vi "getHWConfig.vi"(8 "error in (no error)":errorcluster, 11 "HWConfiguration in":refnum<class "HWConfiguration.lvclass">) -> (0 "error out":errorcluster, 3 "HWConfiguration out":refnum<class "HWConfiguration.lvclass">)   [LabVIEW 2009, in "Hardware.lvlib" / "HWControllers.lvlib" / "HWConfiguration.lvclass"]
uses:
  HWConfiguration.lvclass
  HWConfiguration.lvclass/HWConfiguration.ctl
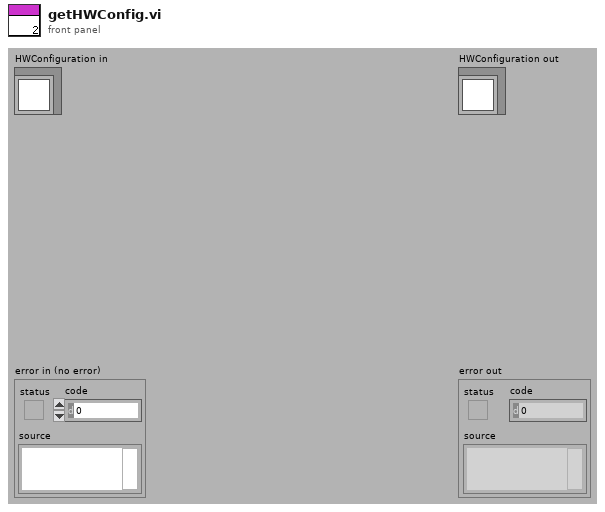
[diagram p1: front panel]
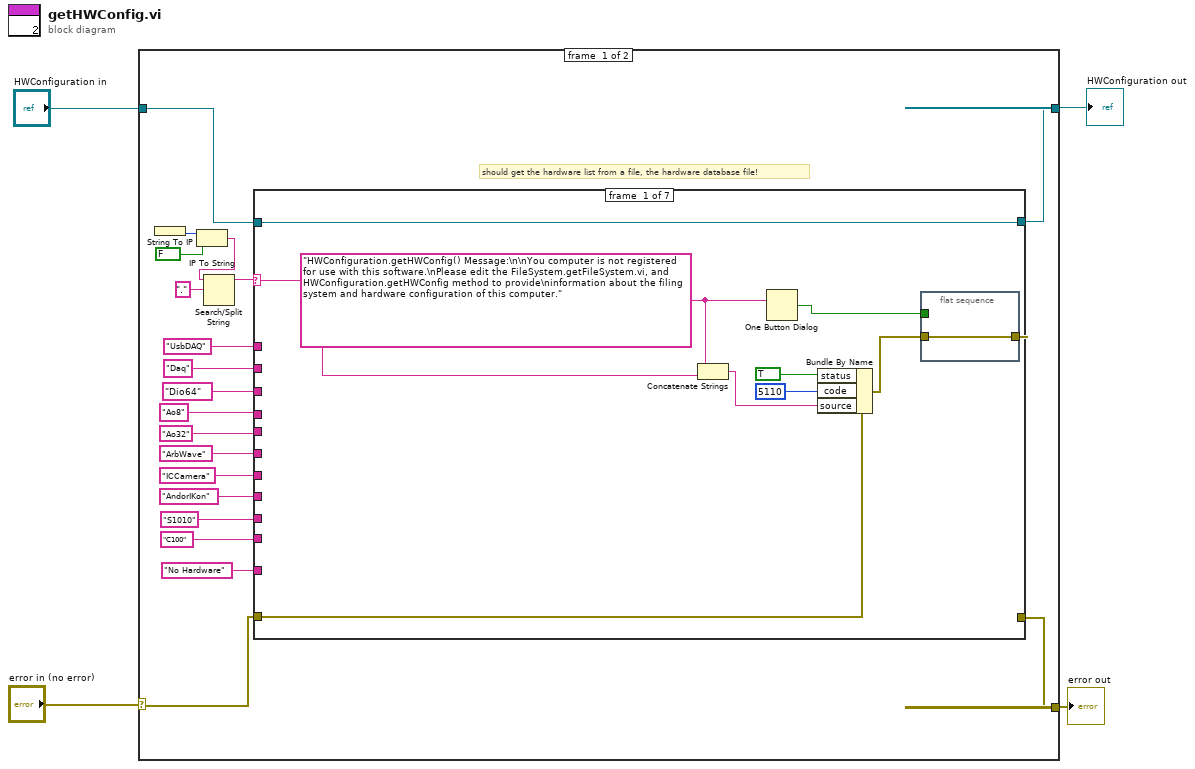
[diagram p0: block diagram]
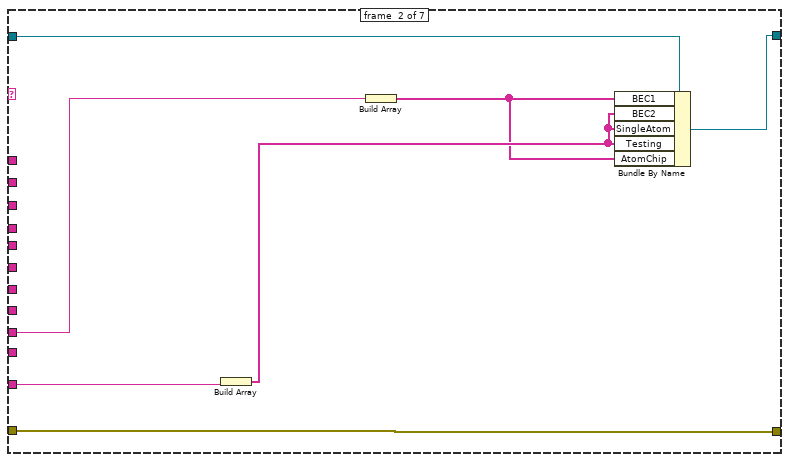
[diagram p2: hidden frame]
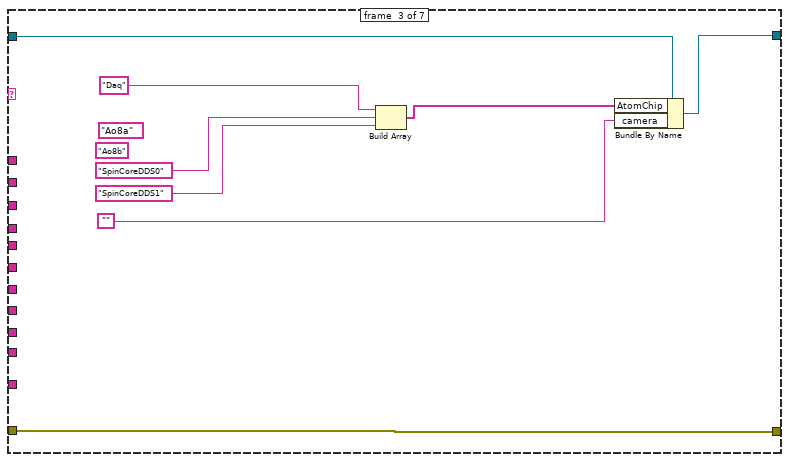
[diagram p3: hidden frame]
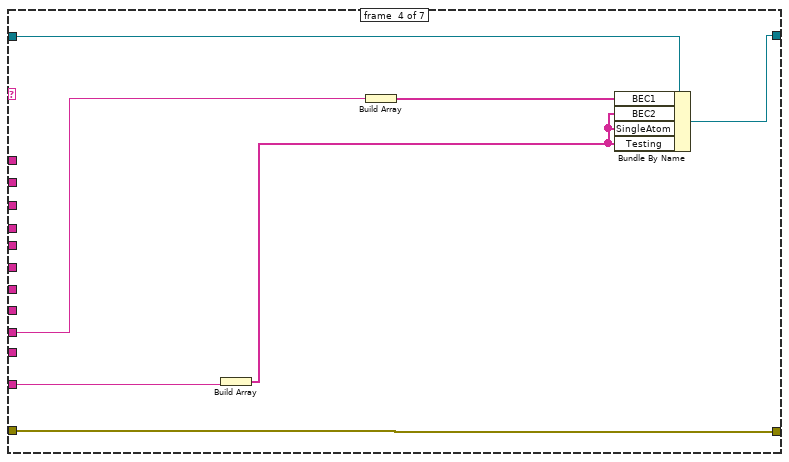
[diagram p4: hidden frame]
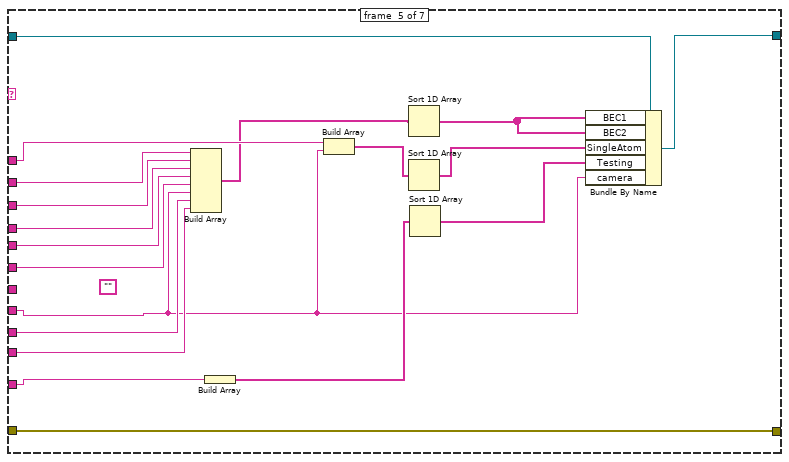
[diagram p5: hidden frame]
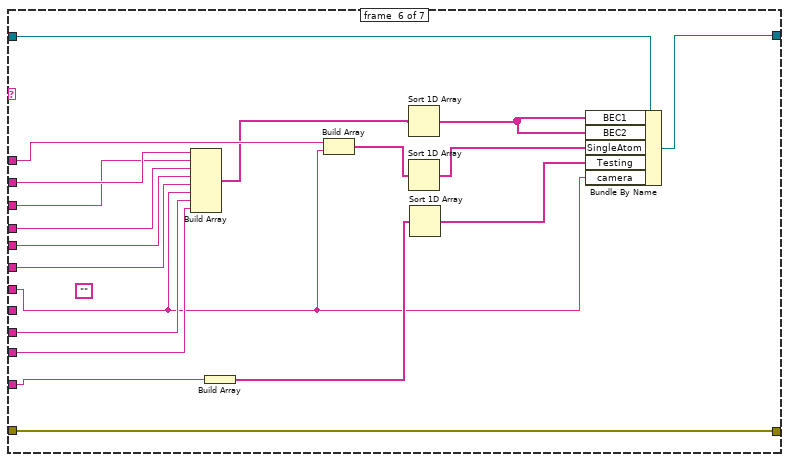
[diagram p6: hidden frame]
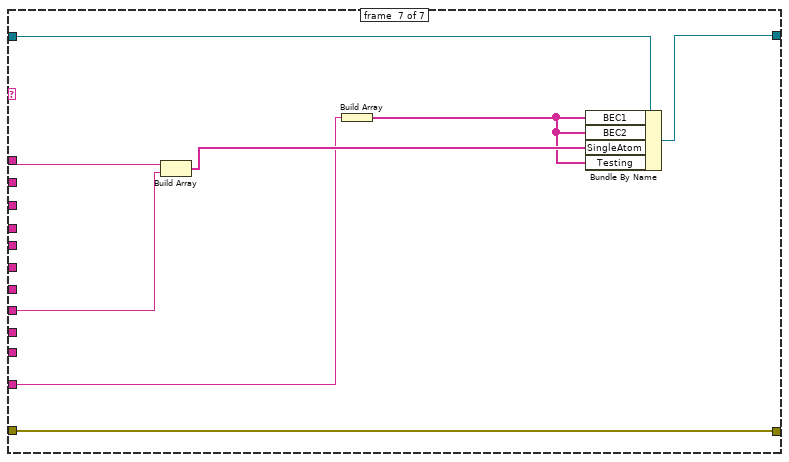
[diagram p7: hidden frame]
diagram:
  n1 = case shown="No Error" "error in (no error)" {
    selector: "error in (no error)" -> [w19 w105]
    tunnel: [w16 w105] -> w3
    tunnel: [w17 w104] -> w1
    tunnel: "HWConfiguration in" -> [w18 w104]
    frame #0 {
      # "should get the hardware list from a file, the hardware database file!"
      n2 = String To IP() -> (0:w23:u32)  [unwired: 1 in]
      n3 = IP To String(1:FALSE, 2:w23) -> (0:w21:string)
      n4 = Search/Split String(string=w21, search string/char (-)=".") -> (substring before match=w20:string)  [unwired: 1 in, 2 out]
      n5 = case shown="\"FCTX52S\"" w20 {
        selector: w20 -> [w28 _ _ _ _ _ _]
        tunnel: w18 -> [w25 w41 w49 w56 w75 w94 w102]
        tunnel: [w25 w40 w48 w55 w74 w93 w101] -> w17
        tunnel: w19 -> [w26 w42 w50 w57 w76 w95 w103]
        tunnel: [w31 w42 w50 w57 w76 w95 w103] -> w16
        tunnel: "UsbDAQ" -> [_ _ _ _ w66 w85 w100]
        tunnel: "Daq" -> [_ _ _ _ w73 w92 _]
        tunnel: "Dio64" -> [_ _ _ _ w59 w77 _]
        tunnel: "Ao8" -> [_ _ _ _ w72 w91 _]
        tunnel: "Ao32" -> [_ _ _ _ w71 w90 _]
        tunnel: "ArbWave" -> [_ _ _ _ w70 w89 _]
        tunnel: "ICCamera" -> [_ _ _ _ _ w78 _]
        tunnel: "AndorIKon" -> [_ _ _ _ w58 _ w99]
        tunnel: "S1010" -> [_ w37 _ w52 w69 w88 _]
        tunnel: "C100" -> [_ _ _ _ w68 w87 _]
        tunnel: "No Hardware" -> [_ w39 _ w54 w67 w86 w96]
        frame #0 {
          w29 = "HWConfiguration.getHWConfig() Message:\n\nYou computer is not registered for use with this software.\nPlease edit the FileSystem.getFileSystem.vi, and HWConfiguration.getHWConfig method to provide\ninformation about the filing system and hardware configuration of this computer."
          n6 = Concatenate Strings(w29, w28) -> (w27:string)
          n7 = One Button Dialog(message=w29) -> (true=w30:bool)  [unwired: 1 in]
          n8 = Bundle By Name(cluster=w26, "status"=TRUE, "code"=5110, "source"=w27) -> (w32:errorcluster)
          n9 = flat-sequence {
            tunnel: w32 -> [w35]
            tunnel: [w35] -> w31
            tunnel: w30 -> [_]
            frame #0 {
            }
          }
        }
        frame #1 {
          n10 = Build Array(w39) -> (w38:string[])
          n11 = Build Array(w37) -> (w36:string[])
          n12 = Bundle By Name(cluster=w41, "BEC1"=w36, "BEC2"=w38, "SingleAtom"=w38, "Testing"=w38, "AtomChip"=w36) -> (w40:refnum<class "HWConfiguration.lvclass">)
        }
        frame #2 {
          (unwired) "Ao8b"
          (unwired) "Ao8a"
          n13 = Build Array("Daq", "SpinCoreDDS0", "SpinCoreDDS1") -> (w45:string[])
          n14 = Bundle By Name(cluster=w49, "AtomChip"=w45, "camera"="") -> (w48:refnum<class "HWConfiguration.lvclass">)
        }
        frame #3 {
          n15 = Build Array(w54) -> (w53:string[])
          n16 = Build Array(w52) -> (w51:string[])
          n17 = Bundle By Name(cluster=w56, "BEC1"=w51, "BEC2"=w53, "SingleAtom"=w53, "Testing"=w53) -> (w55:refnum<class "HWConfiguration.lvclass">)
        }
        frame #4 {
          (unwired) ""
          n18 = Build Array(w73, w59, w72, w71, w70, w58, w69, w68) -> (w65:string[])
          n19 = Build Array(w67) -> (w61:string[])
          n20 = Build Array(w66, w58) -> (w63:string[])
          n21 = Sort 1D Array(array=w65) -> (sorted array=w64:string[])
          n22 = Sort 1D Array(array=w63) -> (sorted array=w62:string[])
          n23 = Sort 1D Array(array=w61) -> (sorted array=w60:string[])
          n24 = Bundle By Name(cluster=w75, "BEC1"=w64, "BEC2"=w64, "SingleAtom"=w62, "Testing"=w60, "camera"=w58) -> (w74:refnum<class "HWConfiguration.lvclass">)
        }
        frame #5 {
          (unwired) ""
          n25 = Build Array(w92, w77, w91, w90, w89, w78, w88, w87) -> (w84:string[])
          n26 = Build Array(w86) -> (w80:string[])
          n27 = Build Array(w85, w78) -> (w82:string[])
          n28 = Sort 1D Array(array=w84) -> (sorted array=w83:string[])
          n29 = Sort 1D Array(array=w82) -> (sorted array=w81:string[])
          n30 = Sort 1D Array(array=w80) -> (sorted array=w79:string[])
          n31 = Bundle By Name(cluster=w94, "BEC1"=w83, "BEC2"=w83, "SingleAtom"=w81, "Testing"=w79, "camera"=w78) -> (w93:refnum<class "HWConfiguration.lvclass">)
        }
        frame #6 {
          n32 = Build Array(w100, w99) -> (w98:string[])
          n33 = Build Array(w96) -> (w97:string[])
          n34 = Bundle By Name(cluster=w102, "BEC1"=w97, "BEC2"=w97, "SingleAtom"=w98, "Testing"=w97) -> (w101:refnum<class "HWConfiguration.lvclass">)
        }
      }
    }
    frame #1 {
    }
  }
  "error out" <- w3
  "HWConfiguration out" <- w1
